vi "Edge Detection Hatch.vi"(7 "error in":errorcluster) -> (27 "error out":errorcluster)   [LabVIEW 2018]
uses:
  <vilib>/vision/driver/IMAQdx.llb/IMAQdx Camera Control Mode.ctl
  <vilib>/userdefined/High Color/IMAQdx.ctl
  <vilib>/vision/Measure.llb/Edge Options.ctl
  <vilib>/vision/Measure.llb/Edge Polarity.ctl
  <vilib>/vision/Measure.llb/Straight Edge Options.ctl
  <vilib>/vision/Measure.llb/Straight Edge Process.ctl
  <vilib>/Analysis/baseanly.llb/Mean (DBL).vi
  <vilib>/Analysis/1siggen.llb/Ramp Pattern by Delta.vi
  <vilib>/vision/NI_Vision_Development_Module.lvlib
  <vilib>/Analysis/NI_AALBase.lvlib
  <vilib>/Analysis/NI_AALPro.lvlib
  <vilib>/vision/driver/NI_Vision_Acquisition_Software.lvlib
  <resource>/objmgr/imaqdx.rc
panel:
  out "Particle Reports (Pixels)":T1(array[cluster]) {"Orientation" format="%.2f"; "Dimensions"."Height" format="%.2f"; "Dimensions"."Width" format="%.2f"; "Center of Mass"."Y" format="%.2f"; "Center of Mass"."X" format="%.2f"; "Bounding Rect"."Bottom" format="%.2f"; "Bounding Rect"."Right" format="%.2f"; "Bounding Rect"."Top" format="%.2f"; "Bounding Rect"."Left" format="%.2f"; "Number of Holes" format="%.2f"; "Area" format="%.2f"}
  out "Centerpoint 3":cluster{dbl, dbl}
  out "Merged Centerpoint":cluster{dbl, dbl}
  out "Centerpoint 2":cluster{dbl, dbl}
  out "Centerpoint":cluster{dbl, dbl}
  out "Image Out 2":T2(plugin-control)
  in  "error in 3":errorcluster
  in  "error in 2":errorcluster
  out "Run time":u32
  out "dX/dt":dbl[](array[numeric])
  out "dY/dt":dbl[](array[numeric])
  out "Vertical Value":cluster{"Ramp Pattern":dbl[], sgl[]}(graph)
  out "Vertical Derivative":T3(graph)
  out "Horizontal Derivative":T3(graph)
  out "Horizontal Value":cluster{"Ramp Pattern":dbl[], sgl[]}(graph)
  out "Image Out":T2(plugin-control)
types:
  T1 = cluster{"Area":dbl, "Number of Holes":dbl, "Bounding Rect":cluster{"Left":dbl, "Top":dbl, "Right":dbl, "Bottom":dbl}, "Center of Mass":cluster{"X":dbl, "Y":dbl}, "Orientation":dbl, "Dimensions":cluster{"Width":dbl, "Height":dbl}}[]
  T2 = typedef "IMAQ Image.ctl" = refnum<image>
  T3 = cluster{"Nth Derivative of P(x)":dbl[], "Ramp Pattern":dbl[]}
  T4 = typedef "IMAQdx.ctl" = refnum<k21>
  T5 = typedef "NI_Vision_Acquisition_Software.lvlib/IMAQdx Camera Control Mode.ctl" = enum32{"Controller", "Listener"}
  T6 = typedef "Image Type" = u32
  T7 = cluster{"Measurement Parameter":i32, "Range Lower Value":dbl, "Range Upper Value":dbl, "Range":bool, "Measurement Type":bool}[]
  T8 = enum32{"AutoM", "Close", "Dilate", "Erode", "Gradient", "Gradient out", "Gradient in", "Hit miss", "Open", "PClose", "POpen", "Thick", "Thin"}
  T9 = typedef "Straight Edge Options.ctl" = cluster{"Number of Lines":i32, "Type":T10, "Min. Score":dbl, "Max. Score":dbl, "Orientation":dbl, "Angle Range":dbl, "Angle Tolerance":dbl, "Step Size":u32, "Min. SNR (db)":dbl, "Min. Points (%)":dbl, "Hough Iterations":i32}
  T10 = typedef "Straight Edge Process.ctl" = enum32{"First Edge Rake", "Best Edge Rake", "Hough Edge Rake", "First Edge Projection", "Best Edge Projection"}
  T11 = typedef "Edge Options.ctl" = cluster{"Edge Polarity":T12, "Kernel Size":u32, "Width":u32, "Minimum Edge Strength":sgl, "Interpolation Type":enum32{"Zero Order", "Bilinear", "Quadratic", "Cubic", "Bilinear Fixed"}, "Data Processing Method":enum32{"Average", "Median"}}
  T12 = typedef "Edge Polarity.ctl" = u32
  T13 = typedef "ROI Descriptor" = cluster{"Global Rectangle":i32[], "Contours":cluster{"ID":enum32{"External", "Internal"}, "Type":u32, "Coordinates":i32[]}[]}
  T14 = cluster{"histogram":u32[], "Minimal Value":sgl, "Maximal Value":sgl, "Starting Value":sgl, "Interval Width":sgl, "Mean Value":sgl, "Standard  Variation":sgl, "Area (pixels)":i32}
  T15 = typedef "Search Line.ctl" = cluster{"Start Point":cluster{"X":sgl, "Y":sgl}, "End Point":cluster{"X":sgl, "Y":sgl}, "Edge Info":T16[], "Edge Map":dbl[], "Calibration Valid":bool}
  T16 = typedef "Edge New.ctl" = cluster{"Location (Pixel)":cluster{"X":sgl, "Y":sgl}, "Location (Real-World)":cluster{"X":sgl, "Y":sgl}, "Distance (Pixel)":dbl, "Distance (Real-World)":dbl, "Strength":dbl, "Noise":dbl, "Rising?":bool}
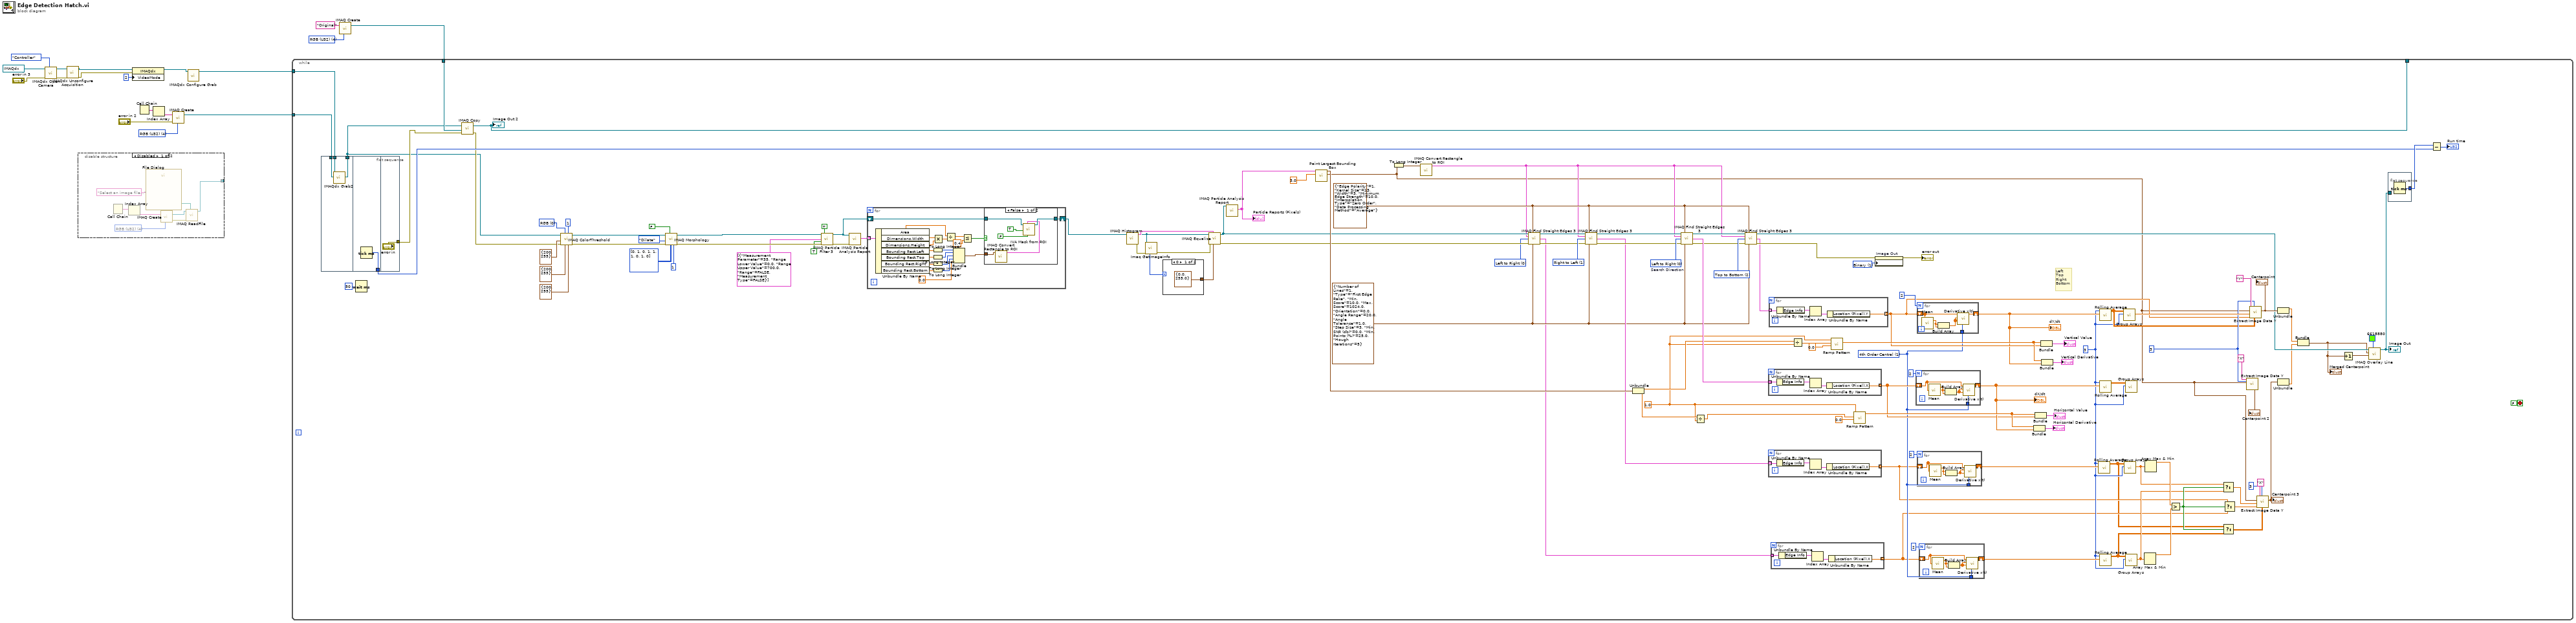
[diagram p0: block diagram]
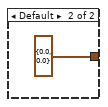
[diagram p4: hidden frame]
diagram:
  w6 = T6 4 items=["Grayscale (U8)", "Grayscale (I16)", "Grayscale (SGL)", "Complex (CSG)", "RGB (U32)", "HSL (U32)", "RGB (U64)", "Grayscale (U16)"] ("Image Type")
  w18 = T6 4 items=["Grayscale (U8)", "Grayscale (I16)", "Grayscale (SGL)", "Complex (CSG)", "RGB (U32)", "HSL (U32)", "RGB (U64)", "Grayscale (U16)"] ("Image Type")
  n1 = call <vilib>:"IMAQdx Open Camera.vi"("Camera Control Mode"=IMAQdx_Camera_Control_Mode."Controller", "error in"="error in 3", "Session In"=T4 "cam1") -> ("error out"=w12:errorcluster, "Session Out"=w13:T4)  [unwired: 7 in]
  n2 = call <vilib>:"IMAQdx Unconfigure Acquisition.vi"("error in"=w12, "Session In"=w13) -> ("error out"=w15:errorcluster, "Session Out"=w14:T4)  [unwired: 8 in]
  n3 = disable-structure shown="Disabled" {
    disable-tunnel: [w26 _] -> _
    frame Disabled {
      w19 = T6 4 items=["Grayscale (U8)", "Grayscale (I16)", "Grayscale (SGL)", "Complex (CSG)", "RGB (U32)", "HSL (U32)", "RGB (U64)", "Grayscale (U16)"] ("Image Type")
      n4 = Call Chain() -> (call chain=w22:string[])
      n5 = Index Array(array=w22) -> (element=w23:string)  [unwired: 1 in]
      n6 = call "File Dialog"("prompt"="Select an image file...") -> ("selected path"=w24:path)  [unwired: 6 in, 8 out]
      n7 = call "IMAQ Create"("Image Name"=w23, "Image Type"=w19) -> ("New Image"=w20:T2, "error out"=w21:errorcluster)  [unwired: 2 in, 1 out]
      n8 = call "IMAQ ReadFile"("File Path"=w24, "error in (no error)"=w21, "Image"=w20) -> ("Image Out"=w26:T2)  [unwired: 2 in, 6 out]
    }
    frame Enabled {
    }
  }
  n9 = property class="IMAQdx"(reference=w14, error in=w15, "VideoMode"=u32 2) -> (reference out=w11:T4)  [unwired: 1 out]
  n10 = Call Chain() -> (call chain=w8:string[])
  n11 = Index Array(array=w8) -> (element=w7:string)  [unwired: 1 in]
  n12 = call "IMAQ Create"("Image Name"=w7, "Image Type"=w6, "error in (no error)"="error in 2") -> ("New Image"=w2:T2)  [unwired: 1 in, 2 out]
  n13 = call <vilib>:"IMAQdx Configure Grab.vi"("Session In"=w11) -> ("Session Out"=w1:T4)  [unwired: 9 in, 1 out]
  n14 = call "IMAQ Create"("Image Name"="Original", "Image Type"=w18) -> ("New Image"=w16:T2)  [unwired: 2 in, 2 out]
  n15 = while {
    tunnel: w16 -> [w107]
    tunnel: [w96] -> _
    tunnel: w2 -> [w83]
    tunnel: w1 -> [w82]
    stop <- FALSE ("stop") stop-if-true
    w45 = u32 0 items=["Left to Right", "Right to Left", "Top to Bottom", "Bottom to Top"] ("Search Direction")
    w61 = u32 1 items=["Left to Right", "Right to Left", "Top to Bottom", "Bottom to Top"] ("Search Direction")
    w47 = T9 {"Number of Lines"=1, "Type"=enum."First Edge Rake", "Min. Score"=10.0, "Max. Score"=1024.0, "Orientation"=0.0, "Angle Range"=20.0, "Angle Tolerance"=1.0, "Step Size"=3, "Min. SNR (db)"=0.0, "Min. Points (%)"=25.0, "Hough Iterations"=5} ("Line Options")
    w48 = T11 {"Edge Polarity"=1, "Kernel Size"=13, "Width"=3, "Minimum Edge Strength"=10.0, "Interpolation Type"=enum."Zero Order", "Data Processing Method"=enum."Average"} ("Edge Options")
    w70 = 3 ("Detector Interval")
    w43 = 3 ("length")
    w53 = u16 1 items=["2nd Order Central", "4th Order Central", "Forward", "Backward"] ("method")
    w118 = u32 2 items=["Left to Right", "Right to Left", "Top to Bottom", "Bottom to Top"] ("Search Direction")
    w113 = 1.0 ("delta")
    w122 = u32 1 items=["Grayscale", "Binary", "Gradient", "Rainbow", "Temperature", "User Defined", "Binary 16 Bit", "Gradient 16 Bit", "Rainbow 16 Bit", "Temperature 16 Bit", "User Defined 16 Bit"] ("Palette Type")
    w124 = u32 0 items=["Left to Right", "Right to Left", "Top to Bottom", "Bottom to Top"]  # Search Direction
    w144 = u16 0 items=["RGB", "HSL", "HSV", "HSI"] ("Color Mode")
    # "Left\nTop\nRight\nBottom"
    n16 = flat-sequence {
      tunnel: w83 -> [w212]
      tunnel: w82 -> [w211]
      tunnel: [w210] -> w81
      tunnel: [w213] -> w111
      tunnel: ["error in"] -> w103
      frame #0 {
        n17 = call <vilib>:"IMAQdx Grab2.vi"("Image In"=w212, "Session In"=w211) -> ("Image Out"=w210:T2)  [unwired: 6 in, 3 out]
      }
      frame #1 {
        n18 = Tick Count (ms)() -> (millisecond timer value=w213:u32)
      }
      frame #2 {
      }
    }
    n19 = Wait (ms)(milliseconds to wait=u32 50) -> ()  [unwired: 1 out]
    n20 = call "IMAQ Copy"("error in (no error)"=w103, "Image Dst"=w107, "Image Src"=w81) -> ("error out"=w106:errorcluster, "Image Dst Out"=w96:T2)  [unwired: 3 in]
    "Image Out 2" <- w96
    n21 = call "IMAQ ColorThreshold"("Blue or Luma or Val or Inten Range"=cluster{"Lower value":i32, "Upper value":i32} {"Lower value"=200, "Upper value"=255}, "Replace Value"=1, "Green or Sat Range"=cluster{"Lower value":i32, "Upper value":i32} {"Lower value"=200, "Upper value"=255}, "Color Mode"=w144, "error in (no error)"=w106, "Red or Hue Range"=cluster{"Lower value":i32, "Upper value":i32} {"Lower value"=200, "Upper value"=255}, "Image Src"=w81) -> ("error out"=w140:errorcluster, "Image Dst Out"=w135:T2)  [unwired: 1 in, 2 out]
    n22 = call "IMAQ Morphology"("Number of iterations (1)"=1, "Structuring Element"=i32[][] [[0, 1, 0], [1, 1, 1], [0, 1, 0]], "Square/Hexa (Square)"=FALSE, "error in (no error)"=w140, "Operation"=T8."Dilate", "Image Src"=w135) -> ("error out"=w134:errorcluster, "Image Dst Out"=w131:T2)  [unwired: 1 in, 3 out]
    n23 = call "IMAQ Particle Filter 3"("Image Src"=w131, "Connectivity 4/8 (8)"=TRUE, "Selection Values"=T7 [{"Measurement Parameter"=35, "Range Lower Value"=0.0, "Range Upper Value"=700.0, "Range"=FALSE, "Measurement Type"=FALSE}], "Keep/Remove Particles (F)"=TRUE ("Keep/Remove Particles"), "error in (no error)"=w134) -> ("Image Dst Out"=w101:T2, "error out"=w105:errorcluster)  [unwired: 4 in, 5 out]
    n24 = call "IMAQ Particle Analysis Report"("error in (no error)"=w105, "Image"=w101) -> ("Particle Reports (Pixels)"=w100:T1)  [unwired: 4 in, 5 out]
    n25 = for {
      tunnel: w100 -> [w201] mode=indexing
      shift-right: [w193] -> w102
      shift-left: w101 -> [w194]
      n26 = Unbundle By Name(w201) -> ("Area"=w198:dbl, "Dimensions.Width"=w200:dbl, "Dimensions.Height"=w199:dbl, "Bounding Rect.Left"=w191:dbl, "Bounding Rect.Top"=w190:dbl, "Bounding Rect.Right"=w189:dbl, "Bounding Rect.Bottom"=w188:dbl)
      n27 = To Long Integer(number=w191) -> (32bit integer=w187:i32)
      n28 = To Long Integer(number=w190) -> (32bit integer=w186:i32)
      n29 = To Long Integer(number=w189) -> (32bit integer=w185:i32)
      n30 = To Long Integer(number=w188) -> (32bit integer=w184:i32)
      n31 = Multiply(x=w200, y=w199) -> (x*y=w197:dbl)
      n32 = Divide(x=w198, y=w197) -> (x/y=w196:dbl)
      n33 = Bundle(w187, w186, w185, w184, 0.0) -> (w183:cluster{i32, i32, i32, i32, dbl})  [unwired: 1 in]
      n34 = Less Or Equal?(x=w196, y=0.4) -> (x <= y?=w192:bool)
      n35 = case shown="False" w192 {
        tunnel: w194 -> [w204 w208]
        tunnel: [w203 w208] -> w193
        tunnel: w183 -> [w207 _]
        frame False {
          n36 = call "IMAQ Convert Rectangle to ROI"("Rectangle"=w207) -> ("ROI Descriptor"=w202:T13)  [unwired: 8 in, 1 out]
          n37 = call <vilib>:"IVA Mask from ROI.vi"("Shrink"=FALSE, "ROI Descriptor"=w202, "Out / In"=TRUE, "Image Src"=w204) -> ("Image Out"=w203:T2)  [unwired: 1 in, 6 out]
        }
        frame True {
        }
      }
    }
    n38 = call "IMAQ Histogram"("Image"=w102) -> ("error out"=w127:errorcluster, "Histogram Report"=w129:T14)  [unwired: 4 in, 5 out]
    n39 = call "Imaq GetImageInfo"("error in (no error)"=w127, "Image"=w102) -> ("error out"=w126:errorcluster, "Image Type"=w128:T6)  [unwired: 8 out]
    n40 = case shown="0" w128 {
      tunnel: [cluster{"Minimum":sgl, "Maximum":sgl} {"Minimum"=0.0, "Maximum"=255.0} ("Range") cluster{"Minimum":sgl, "Maximum":sgl} {"Minimum"=0.0, "Maximum"=0.0} ("Range")] -> w125
      frame 0 {
      }
      frame Default {
      }
    }
    n41 = call "IMAQ Equalize"("Range"=w125, "Histogram Report"=w129, "error in (no error)"=w126, "Image Src"=w102) -> ("error out"=w50:errorcluster, "Image Dst Out"=w52:T2)  [unwired: 2 in, 4 out]
    n42 = call "IMAQ Particle Analysis Report"("Image"=w52) -> ("Particle Reports (Pixels)"=w99:T1)  [unwired: 5 in, 5 out]
    "Particle Reports (Pixels)" <- w99
    n43 = call "Paint Largest Bounding Box.vi"("Border Width"=3.0, "Particle Reports (Pixels)"=w99) -> ("Bounding Box"=w30:cluster{dbl, dbl, dbl, dbl, dbl}, "Dimensions"=w97:cluster{dbl, dbl})  [unwired: 8 in]
    n44 = To Long Integer(number=w30) -> (32bit integer=w120:cluster{i32, i32, i32, i32, i32})
    n45 = call "IMAQ Convert Rectangle to ROI"("Rectangle"=w120) -> ("ROI Descriptor"=w46:T13)  [unwired: 8 in, 1 out]
    n46 = call "IMAQ Find Straight Edges 3"("Image"=w52, "Edge Options"=w48, "ROI Descriptor"=w46, "Search Direction"=w45, "error in (no error)"=w50, "Line Options"=w47) -> ("Image (duplicate)"=w51:T2, "Search Lines Information"=w44:T15[], "error out"=w49:errorcluster)  [unwired: 1 in, 6 out]
    n47 = call "IMAQ Find Straight Edges 3"("Image"=w51, "Edge Options"=w48, "ROI Descriptor"=w46, "Search Direction"=w61, "error in (no error)"=w49, "Line Options"=w47) -> ("Image (duplicate)"=w63:T2, "Search Lines Information"=w60:T15[], "error out"=w62:errorcluster)  [unwired: 1 in, 6 out]
    n48 = Unbundle(w97) -> (w114:dbl, w115:dbl)
    n49 = call "IMAQ Find Straight Edges 3"("Image"=w63, "Edge Options"=w48, "ROI Descriptor"=w46, "Search Direction"=w124, "error in (no error)"=w62, "Line Options"=w47) -> ("Image (duplicate)"=w104:T2, "Search Lines Information"=w121:T15[], "error out"=w80:errorcluster)  [unwired: 1 in, 6 out]
    n50 = Divide(x=w115, y=w113) -> (x/y=w116:dbl)
    n51 = call "IMAQ Find Straight Edges 3"("Image"=w104, "Edge Options"=w48, "ROI Descriptor"=w46, "Search Direction"=w118, "error in (no error)"=w80, "Line Options"=w47) -> ("Image (duplicate)"=w73:T2, "Search Lines Information"=w117:T15[], "error out"=w119:errorcluster)  [unwired: 1 in, 6 out]
    n52 = for {
      tunnel: w121 -> [w181] mode=indexing
      tunnel: [w178] -> w58 mode=indexing
      n53 = Unbundle By Name(w181) -> ("Edge Info"=w180:T16[])
      n54 = Index Array(array=w180) -> (element=w179:T16)  [unwired: 1 in]
      n55 = Unbundle By Name(w179) -> ("Location (Pixel).X"=w178:sgl)
    }
    n56 = for {
      tunnel: w60 -> [w163] mode=indexing
      tunnel: [w160] -> w37 mode=indexing
      n57 = Unbundle By Name(w163) -> ("Edge Info"=w162:T16[])
      n58 = Index Array(array=w162) -> (element=w161:T16)  [unwired: 1 in]
      n59 = Unbundle By Name(w161) -> ("Location (Pixel).X"=w160:sgl)
    }
    n60 = for {
      tunnel: w117 -> [w177] mode=indexing
      tunnel: [w174] -> w67 mode=indexing
      n61 = Unbundle By Name(w177) -> ("Edge Info"=w176:T16[])
      n62 = Index Array(array=w176) -> (element=w175:T16)  [unwired: 1 in]
      n63 = Unbundle By Name(w175) -> ("Location (Pixel).Y"=w174:sgl)
    }
    n64 = for {
      tunnel: w44 -> [w154] mode=indexing
      tunnel: [w151] -> w36 mode=indexing
      n65 = Unbundle By Name(w154) -> ("Edge Info"=w153:T16[])
      n66 = Index Array(array=w153) -> (element=w152:T16)  [unwired: 1 in]
      n67 = Unbundle By Name(w152) -> ("Location (Pixel).X"=w151:sgl)
    }
    n68 = Divide(x=w114, y=w113) -> (x/y=w88:dbl)
    n69 = call-poly <vilib>:"Ramp Pattern.vi"("start"=0.0, "end"=w88, "delta"=w113) -> ("Ramp Pattern"=w85:dbl[])  [unwired: 6 in, 2 out]
    n70 = call-poly <vilib>:"Ramp Pattern.vi"("start"=0.0, "end"=w116, "delta"=w113) -> ("Ramp Pattern"=w92:dbl[])  [unwired: 6 in, 2 out]
    n71 = property on="Image Out" class="ImageControl"(error in=w119, "Palette:Palette Type"=w122) -> (error out=→"error out":errorcluster)  [unwired: 1 in, 1 out]
    n72 = for {
      N: 2 -> [_]
      tunnel: w53 -> [w172]
      shift-right: [w173] -> w84
      shift-left: w58 -> [w171]
      n73 = call-poly <vilib>:"Mean.vi"("X"=w171) -> ("mean"=w170:dbl)  [unwired: 1 out]
      n74 = Build Array(w170, w170) -> (w169:dbl[])
      n75 = call <vilib>:"Derivative x(t).vi"("method"=w172, "Final Condition"=w169, "Initial Condition"=w169, "X"=w171) -> ("dX/dt"=w173:dbl[])  [unwired: 6 in, 1 out]
    }
    "dX/dt" <- w84
    n76 = for {
      N: 2 -> [_]
      tunnel: w53 -> [w158]
      shift-right: [w159] -> w59
      shift-left: w37 -> [w157]
      n77 = call-poly <vilib>:"Mean.vi"("X"=w157) -> ("mean"=w156:dbl)  [unwired: 1 out]
      n78 = Build Array(w156, w156) -> (w155:dbl[])
      n79 = call <vilib>:"Derivative x(t).vi"("method"=w158, "Final Condition"=w155, "Initial Condition"=w155, "X"=w157) -> ("dX/dt"=w159:dbl[])  [unwired: 6 in, 1 out]
    }
    n80 = for {
      N: 2 -> [_]
      tunnel: w53 -> [w168]
      shift-right: [w165] -> w66
      shift-left: w67 -> [w164]
      n81 = call-poly <vilib>:"Mean.vi"("X"=w164) -> ("mean"=w167:dbl)  [unwired: 1 out]
      n82 = Build Array(w167, w167) -> (w166:dbl[])
      n83 = call <vilib>:"Derivative x(t).vi"("method"=w168, "Final Condition"=w166, "Initial Condition"=w166, "X"=w164) -> ("dX/dt"=w165:dbl[])  [unwired: 6 in, 1 out]
    }
    "dY/dt" <- w66
    n84 = for {
      N: 2 -> [_]
      tunnel: w53 -> [w149]
      shift-right: [w150] -> w54
      shift-left: w36 -> [w148]
      n85 = call-poly <vilib>:"Mean.vi"("X"=w148) -> ("mean"=w147:dbl)  [unwired: 1 out]
      n86 = Build Array(w147, w147) -> (w146:dbl[])
      n87 = call <vilib>:"Derivative x(t).vi"("method"=w149, "Final Condition"=w146, "Initial Condition"=w146, "X"=w148) -> ("dX/dt"=w150:dbl[])  [unwired: 6 in, 1 out]
    }
    n88 = Bundle("Ramp Pattern"=w92, "dX/dt"=w84) -> (→"Horizontal Derivative":cluster{"Ramp Pattern":dbl[], "dX/dt":dbl[]})  [unwired: 1 in]
    n89 = Bundle("Ramp Pattern"=w92, w58) -> (→"Horizontal Value":cluster{"Ramp Pattern":dbl[], sgl[]})  [unwired: 1 in]
    n90 = Bundle("Ramp Pattern"=w85, w67) -> (→"Vertical Value":cluster{"Ramp Pattern":dbl[], sgl[]})  [unwired: 1 in]
    n91 = Bundle("Ramp Pattern"=w85, "dX/dt"=w66) -> (→"Vertical Derivative":cluster{"Ramp Pattern":dbl[], "dX/dt":dbl[]})  [unwired: 1 in]
    n92 = call "Rolling Average.vi"("Filtered X"=w59, "Subset Length"=w43) -> ("Averaged Values"=w35:dbl[][])  [unwired: 9 in]
    n93 = call "Rolling Average.vi"("Filtered X"=w66, "Subset Length"=w43) -> ("Averaged Values"=w65:dbl[][])  [unwired: 9 in]
    n94 = call "Rolling Average.vi"("Filtered X"=w84, "Subset Length"=w43) -> ("Averaged Values"=w57:dbl[][])  [unwired: 9 in]
    n95 = call "Rolling Average.vi"("Filtered X"=w54, "Subset Length"=w43) -> ("Averaged Values"=w34:dbl[][])  [unwired: 9 in]
    n96 = call "Group Arrays.vi"("length"=w43, "Averaged Values"=w65) -> ("Array"=w79:dbl[])  [unwired: 9 in]
    n97 = call "Group Arrays.vi"("length"=w43, "Averaged Values"=w35) -> ("Array"=w39:dbl[])  [unwired: 9 in]
    n98 = call "Group Arrays.vi"("length"=w43, "Averaged Values"=w57) -> ()  [unwired: 9 in, 1 out]
    n99 = call "Group Arrays.vi"("length"=w43, "Averaged Values"=w34) -> ("Array"=w38:dbl[])  [unwired: 9 in]
    n100 = Array Max & Min(array=w38) -> (max value=w41:dbl)  [unwired: 3 out]
    n101 = Array Max & Min(array=w39) -> (max value=w42:dbl)  [unwired: 3 out]
    n102 = Greater?(x=w42, y=w41) -> (0:w40:bool)
    n103 = Select(t=w39, s=w40, f=w38) -> (s? t:f=w33:dbl[])
    n104 = Select(t=w35, s=w40, f=w34) -> (s? t:f=w31:dbl[][])
    n105 = Select(t=w37, s=w40, f=w36) -> (s? t:f=w32:sgl[])
    n106 = call "Extract Image Data Y.vi"("Detector Interval"=w70, "Bounding Box"=w30, "String"="X") -> ("Centerpoint"=→"Centerpoint 2":cluster{dbl, dbl})  [unwired: 8 in]
    n107 = call "Extract Image Data Y.vi"("Averaged Values"=w65, "Detector Interval"=w70, "Original values"=w67, "Grouped Arrays"=w79, "Bounding Box"=w30, "String"="Y") -> ("Centerpoint"=w76:cluster{dbl, dbl})  [unwired: 5 in]
    "Centerpoint" <- w76
    n108 = call "Extract Image Data Y.vi"("Averaged Values"=w31, "Detector Interval"=3, "Original values"=w32, "Grouped Arrays"=w33, "Bounding Box"=w30, "String"="X") -> ("Centerpoint"=w27:cluster{dbl, dbl})  [unwired: 5 in]
    "Centerpoint 3" <- w27
    n109 = Unbundle(w76) -> (w69:dbl)  [unwired: 1 out]
    n110 = Unbundle(w27) -> (w68:dbl)  [unwired: 1 out]
    n111 = Bundle(w69, w68) -> (w72:cluster{dbl, dbl})  [unwired: 1 in]
    "Merged Centerpoint" <- w72
    n112 = Increment(x=w72) -> (x+1=w71:cluster{dbl, dbl})
    n113 = call "IMAQ Overlay Line"("Color"=u32 6618880, "End Point"=w71, "Start Point"=w72, "Image"=w73) -> ("Image Out"=w64:T2)  [unwired: 6 in, 1 out]
    "Image Out" <- w64
    n114 = flat-sequence {
      tunnel: [w209] -> w112
      tunnel: w64 -> [_]
      frame #0 {
        n115 = Tick Count (ms)() -> (millisecond timer value=w209:u32)
      }
    }
    n116 = Subtract(x=w112, y=w111) -> (x-y=→"Run time":u32)
  }
